vi "Testing (DVR).vi"(8 "error in":errorcluster, 11 "Data Value Reference in":refnum<data-value>) -> (0 "error out":errorcluster, 3 "Data Value Reference out":refnum<data-value>)   [LabVIEW 2016, in "Retrieve and Visualize.lvclass"]
uses:
  Retrieve and Visualize.lvclass
  <userlib>/LevyLab/XY Utilities/subVIs/Multiply float (multiple).vi
  <userlib>/LevyLab/XY Utilities/xy_utilities.lvlib
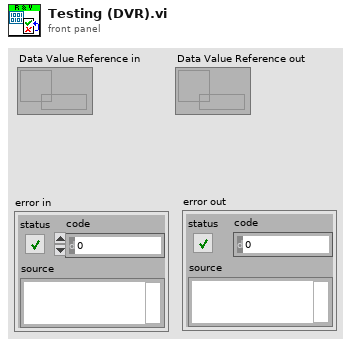
[diagram p1: front panel]
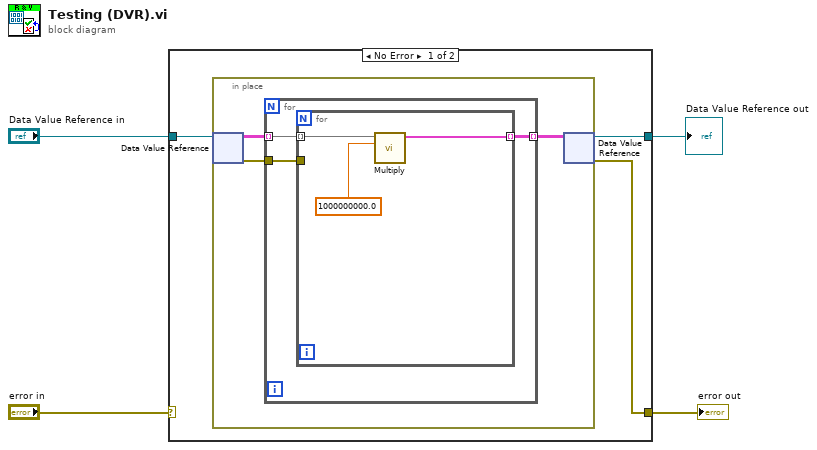
[diagram p0: block diagram]
diagram:
  n1 = case shown="No Error" "error in" {
    selector: "error in" -> [_ w18]
    tunnel: [w7 w17] -> w4
    tunnel: "Data Value Reference in" -> [w6 w17]
    tunnel: [w5 w18] -> w2
    frame No Error {
      n2 = in-place {
        n3 = in-place-dvr #1(w6) -> (w10:cluster{dbl[], dbl[]}[][][], w9:errorcluster)
        n4 = for {
          tunnel: w10 -> [w13] mode=indexing
          tunnel: w9 -> [w12]
          tunnel: [w11] -> w8 mode=indexing
          n5 = for {
            tunnel: w13 -> [w16] mode=indexing
            tunnel: w12 -> [_]
            tunnel: [w15] -> w11 mode=indexing
            n6 = call-poly <userlib>:"Multiply.vi"("x (1)"=1000000000.0, "XY-data"=w16) -> ("XY-data out"=w15:cluster{"X-array":dbl[], "Y-array":dbl[]}[])  [unwired: 8 in, 1 out]
          }
        }
        n7 = in-place-dvr #1(w8) -> (w7:refnum<data-value>, w5:errorcluster)
      }
    }
    frame Error {
    }
  }
  "Data Value Reference out" <- w4
  "error out" <- w2
